vi "StreamEngine.GetNextStreamState.vi"(8 "error in (no error)":errorcluster, 9 "Bus State":T3, 11 "Cmd Q":refnum<queue>) -> (0 "error out":errorcluster, 1 "Bus State":T3, 2 "timed out?":bool, 3 "Command Cluster":T1)   [LabVIEW 2025, in "XNET Bus Monitor Client.lvlib"]
uses:
  XNET Bus Monitor Client.lvlib
  Types/StreamEngine.State.ctl
  Types/StreamEngine.CmdQueueData.ctl
  Types/StreamEngine.CmdQueueData.Cmd.ctl
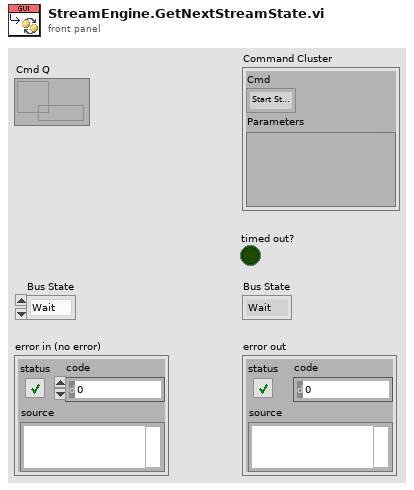
[diagram p1: front panel]
types:
  T1 = typedef "XNET Bus Monitor Client.lvlib/StreamEngine.CmdQueueData.ctl" = cluster{"Cmd":T2, "Parameters":variant}
  T2 = typedef "XNET Bus Monitor Client.lvlib/StreamEngine.CmdQueueData.Cmd.ctl" = enum8{"Start Stream", "Stop Stream", "Exit"}
  T3 = typedef "XNET Bus Monitor Client.lvlib/StreamEngine.State.ctl" = enum8{"Wait", "Start Stream", "Read Stream", "Stop Stream", "Exit"}
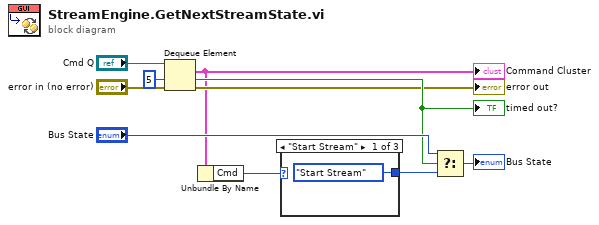
[diagram p0: block diagram]
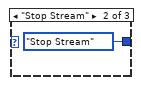
[diagram p2: hidden frame]
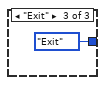
[diagram p3: hidden frame]
diagram:
  n1 = Dequeue Element(queue="Cmd Q", timeout in ms (-1)=5, error in (no error)="error in (no error)") -> (element=w3:T1, timed out?=w7:bool, error out=→"error out":errorcluster)  [unwired: 1 out]
  "Command Cluster" <- w3
  "timed out?" <- w7
  n2 = Unbundle By Name(w3) -> ("Cmd"=w2:T2)
  n3 = case shown="\"Start Stream\"" w2 {
    tunnel: [StreamEngine.State."Start Stream" StreamEngine.State."Stop Stream" StreamEngine.State."Exit"] -> w1
    frame "Start Stream" {
    }
    frame "Stop Stream" {
    }
    frame "Exit" {
    }
  }
  n4 = Select(t="Bus State", s=w7, f=w1) -> (s? t:f=→"Bus State":T3)
